vi "toml_variant_attr_comment.vi"(8 "error in (no error)":errorcluster, 10 "comment":string, 11 "variant in":variant) -> (0 "error out":errorcluster, 3 "variant out":variant)   [LabVIEW 2017]
panel:
  in  "append? (F)":bool
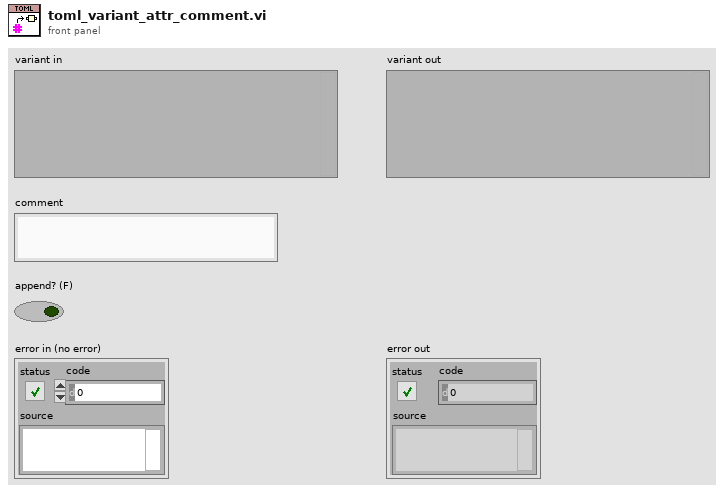
[diagram p1: front panel]
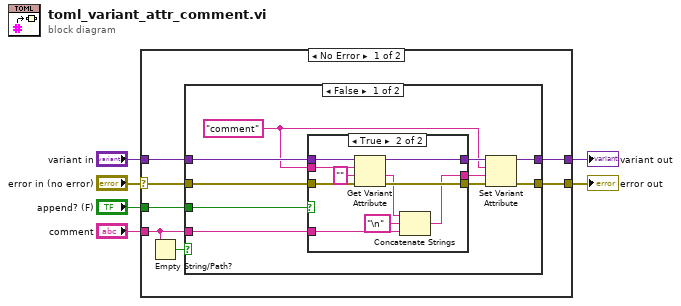
[diagram p0: block diagram]
diagram:
  n1 = case shown="No Error" "error in (no error)" {
    selector: "error in (no error)" -> [w8 w40]
    tunnel: [w9 w40] -> w6
    tunnel: [w13 w39] -> w4
    tunnel: "variant in" -> [w12 w39]
    tunnel: "comment" -> [w11 _]
    tunnel: "append? (F)" -> [w7 _]
    frame No Error {
      n2 = Empty String/Path?(string/path=w11) -> (empty?=w10:bool)
      n3 = case shown="False" w10 {
        tunnel: [w21 w38] -> w13
        tunnel: w12 -> [w17 w38]
        tunnel: w11 -> [w15 _]
        tunnel: [w22 w37] -> w9
        tunnel: w8 -> [w23 w37]
        tunnel: w7 -> [w14 _]
        frame False {
          w16 = "comment" ("name")
          n4 = case shown="True" w14 {
            tunnel: w23 -> [w25 w36]
            tunnel: [w25 w35] -> w20
            tunnel: [w24 w34] -> w19
            tunnel: [w26 w32] -> w18
            tunnel: w17 -> [w24 w29]
            tunnel: w16 -> [_ w28]
            tunnel: w15 -> [w26 w27]
            frame False {
            }
            frame True {
              n5 = Get Variant Attribute(Variant=w29, name=w28, default value (empty Variant)="", error in=w36) -> (duplicate Variant=w34:variant, value=w30:string, error out=w35:errorcluster)  [unwired: 1 out]
              n6 = Concatenate Strings(w30, "\n" ("string"), w27) -> (w32:string)
            }
          }
          n7 = Set Variant Attribute(Variant=w19, name=w16, value=w18, error in=w20) -> (Variant out=w21:variant, error out=w22:errorcluster)  [unwired: 1 out]
        }
        frame True {
        }
      }
    }
    frame Error {
    }
  }
  "error out" <- w6
  "variant out" <- w4
